vi "WFM - BLANK POINT.vi"(11 "Special coordinates (um)":T1) -> (3 "appended array":dbl[](array[numeric]))   [LabVIEW 2017]
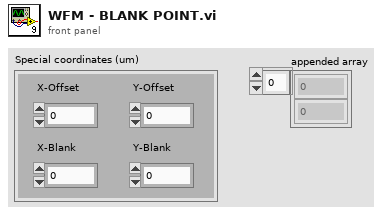
[diagram p1: front panel]
types:
  T1 = cluster{"Y-Offset":dbl, "X-Offset":dbl, "Y-Blank":dbl, "X-Blank":dbl}
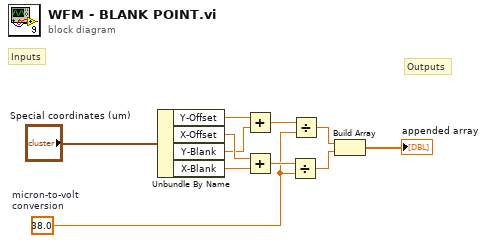
[diagram p0: block diagram]
diagram:
  w4 = 38.0  # micron-to-volt  conversion
  # "Inputs"
  # "Outputs"
  n1 = Unbundle By Name("Special coordinates (um)") -> ("Y-Offset"=w10:dbl, "X-Offset"=w8:dbl, "Y-Blank"=w5:dbl, "X-Blank"=w6:dbl)
  n2 = Add(x=w10, y=w5) -> (x+y=w9:dbl)
  n3 = Add(x=w8, y=w6) -> (x+y=w7:dbl)
  n4 = Divide(x=w7, y=w4) -> (x/y=w3:dbl)
  n5 = Divide(x=w9, y=w4) -> (x/y=w2:dbl)
  n6 = Build Array(w2, w3) -> (→"appended array":dbl[])
